vi "insertTestStandStep.vi"(0 "Sequence File Ref":refnum<k7>, 5 "Step to insert":refnum<k7>, 7 "Step Group":i32(ring)=1 items=["StepGroup_Setup", "StepGroup_Main", "StepGroup_Cleanup"], 9 "index":i32, 11 "error out":errorcluster, 12 "Sequence Name":string="MainSequence") -> (4 "Sequence File Ref(out)":refnum<k7>, 6 "Step to insert (out)":refnum<k7>, 15 "error out":errorcluster)   [LabVIEW 2010]
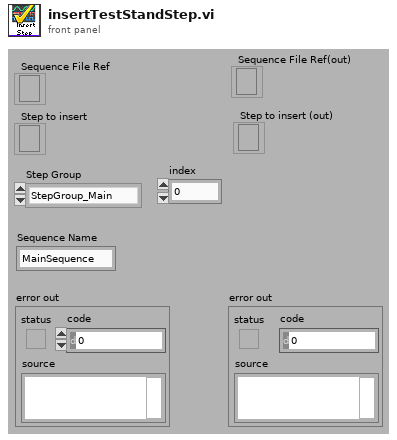
[diagram p1: front panel]
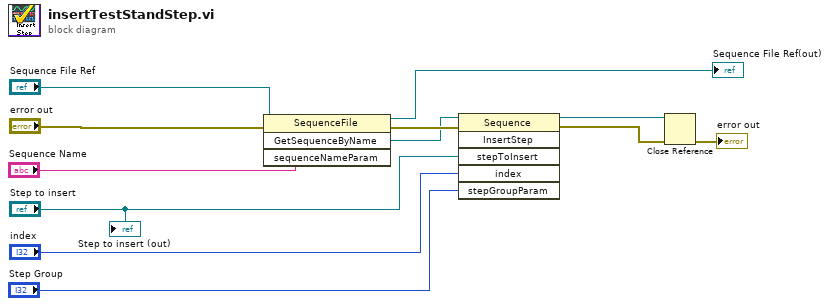
[diagram p0: block diagram]
diagram:
  n1 = invoke class="SequenceFile" method="GetSequenceByName"(reference="Sequence File Ref", error in="error out", "sequenceNameParam"="Sequence Name") -> (reference out=→"Sequence File Ref(out)":refnum<k7>, error out=w12:errorcluster, "GetSequenceByName"=w8:refnum<k7>)  [unwired: 1 in, 1 out]
  n2 = invoke class="Sequence" method="InsertStep"(reference=w8, error in=w12, "stepToInsert"="Step to insert", "index"="index", "stepGroupParam"="Step Group") -> (reference out=w2:refnum<k7>, error out=w3:errorcluster)  [unwired: 1 in, 4 out]
  n3 = Close Reference(reference=w2, error in (no error)=w3) -> (error out=→"error out":errorcluster)
  "Step to insert (out)" <- "Step to insert"
